vi "Homing.vi"(6 "Timeout":i32=60000 caption="Timeout (ms)", 8 "error in (no error)":errorcluster, 11 "FHPP in":refnum<class "FHPP.lvclass">) -> (0 "error out":errorcluster, 1 "TimeOut":bool, 2 "Homed":bool, 3 "FHPP out":refnum<class "FHPP.lvclass">)   [LabVIEW 2022 SP3, in "FHPP.lvclass"]
uses:
  FHPP.lvclass
  <vilib>/GPower/Timing/Library/Remaining/Remaining_ms.vi
  <vilib>/GPower/Timing/GPTiming.lvlib
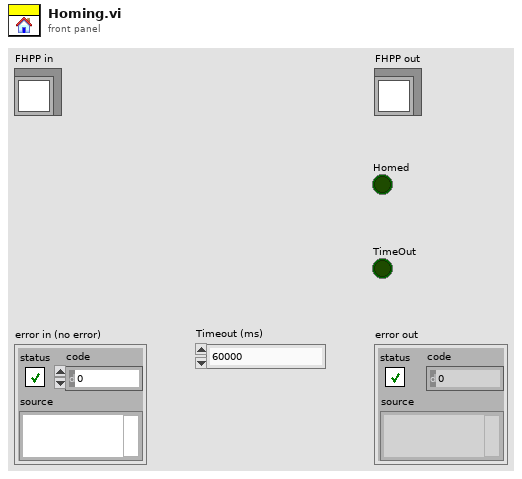
[diagram p1: front panel]
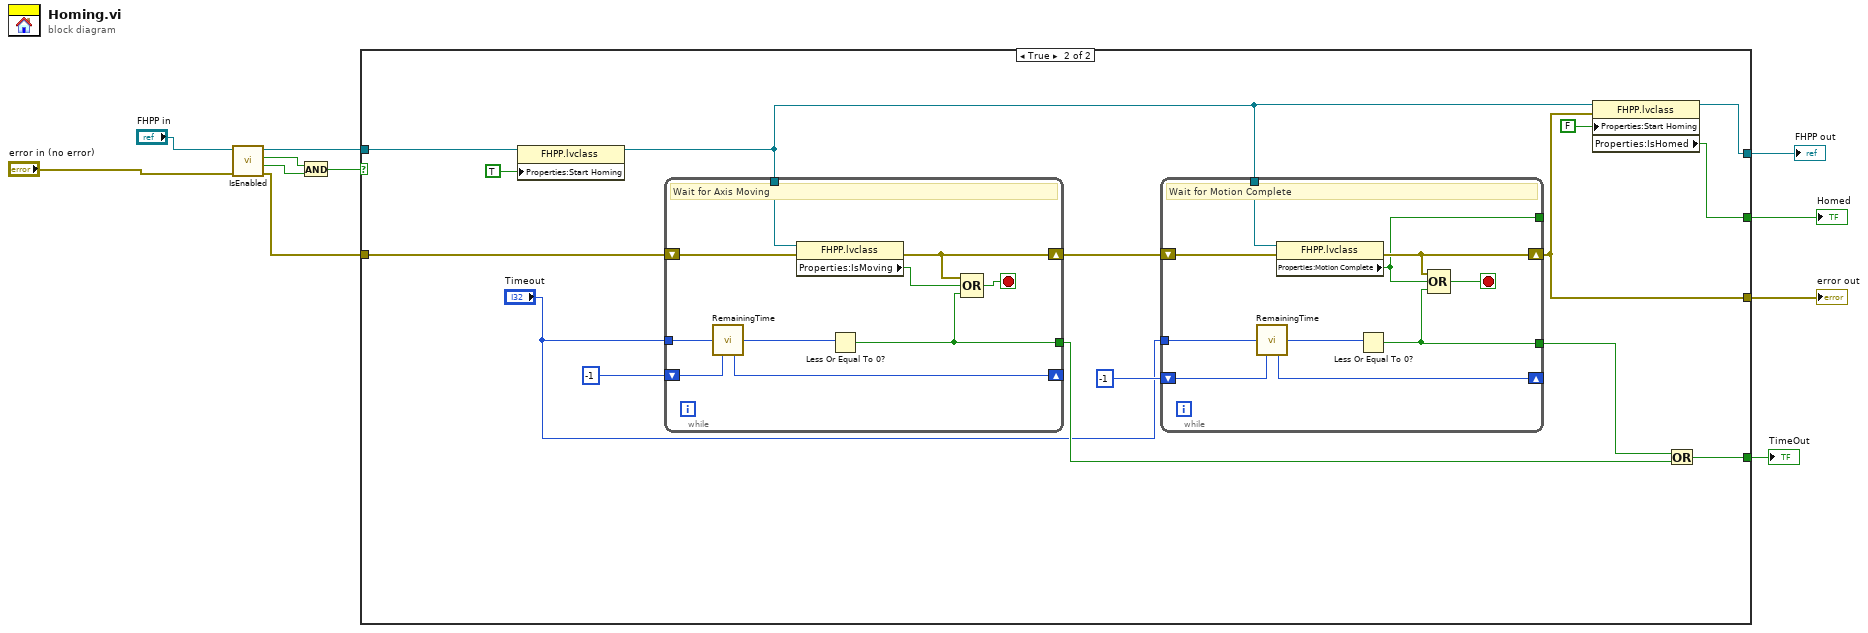
[diagram p0: block diagram]
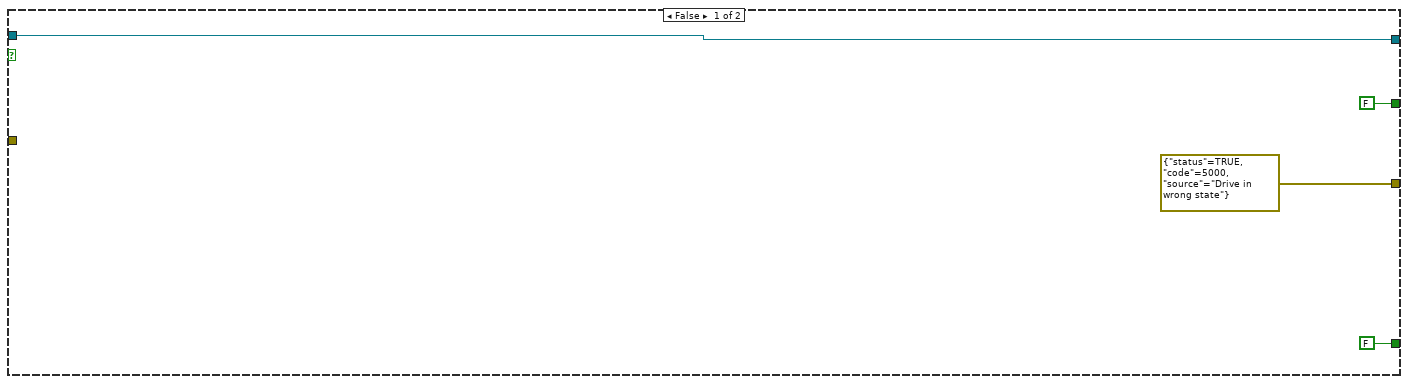
[diagram p2: hidden frame]
diagram:
  n1 = call-dynamic "IsEnabled.vi"("error in (no error)"="error in (no error)", "FHPP in"="FHPP in") -> ("error out"=w7:errorcluster, "Operation Enabled"=w4:bool, "Drive Enabled"=w5:bool, "FHPP out"=w1:refnum<class "FHPP.lvclass">)  [unwired: 6 in]
  n2 = And(x=w5, y=w4) -> (x .and. y?=w6:bool)
  n3 = case shown="True" w6 {
    tunnel: w7 -> [_ w30]
    tunnel: [FALSE w24] -> w9
    tunnel: w1 -> [w15 w23]
    tunnel: [w15 w22] -> w8
    tunnel: [FALSE ("Properties:Motion Complete") w16] -> w3
    tunnel: [errorcluster {"status"=TRUE, "code"=5000, "source"="Drive in wrong state"} ("error out") w17] -> w2
    frame False {
    }
    frame True {
      n4 = property class="FHPP.lvclass"(reference=w23, "Properties:Start Homing"=TRUE ("Start Positioning")) -> (reference out=w20:refnum<class "FHPP.lvclass">)  [unwired: 1 in, 1 out]
      n5 = while {
        tunnel: w20 -> [w50]
        shift-right: [w46] -> w29
        shift-left: w30 -> [w48]
        tunnel: "Timeout" -> [w45]
        shift-right: [w43] -> _
        shift-left: i64 -1 ("Start time in") -> [w44]
        tunnel: [w41] -> w25
        stop <- w47 stop-if-true
        # "Wait for Axis Moving"
        n6 = call-poly <vilib>:"RemainingTime.vi"("Time period target"=w45, "Start time in"=w44) -> ("Remaining time"=w42:i32, "Start time out"=w43:i64)  [unwired: 9 in, 3 out]
        n7 = property class="FHPP.lvclass"(reference=w50, error in=w48) -> (error out=w46:errorcluster, "Properties:IsMoving"=w49:bool)  [unwired: 1 out]
        n8 = Less Or Equal To 0?(x=w42) -> (x <= 0?=w41:bool)
        n9 = Compound Arithmetic op=OR(w46, w49, w41) -> (w47:bool)
      }
      n10 = while {
        tunnel: w20 -> [w40]
        shift-right: [w37] -> w17
        shift-left: w29 -> [w39]
        shift-right: [w35] -> _
        shift-left: i64 -1 ("Start time in") -> [w36]
        tunnel: "Timeout" -> [w34]
        tunnel: [w32] -> w26
        tunnel: [w31] -> _
        stop <- w38 stop-if-true
        # "Wait for Motion Complete"
        n11 = call-poly <vilib>:"RemainingTime.vi"("Time period target"=w34, "Start time in"=w36) -> ("Remaining time"=w33:i32, "Start time out"=w35:i64)  [unwired: 9 in, 3 out]
        n12 = property class="FHPP.lvclass"(reference=w40, error in=w39) -> (error out=w37:errorcluster, "Properties:Motion Complete"=w31:bool)  [unwired: 1 out]
        n13 = Less Or Equal To 0?(x=w33) -> (x <= 0?=w32:bool)
        n14 = Compound Arithmetic op=OR(w37, w31, w32) -> (w38:bool)
      }
      n15 = property class="FHPP.lvclass"(reference=w20, error in=w17, "Properties:Start Homing"=FALSE ("Start Positioning")) -> (reference out=w22:refnum<class "FHPP.lvclass">, "Properties:IsHomed"=w16:bool)  [unwired: 1 out]
      n16 = Or(x=w26, y=w25) -> (x .or. y?=w24:bool)
    }
  }
  "FHPP out" <- w8
  "TimeOut" <- w9
  "Homed" <- w3
  "error out" <- w2
